vi "DeleteOneRecordTo2DListCtrl.vi"(11 "testcaselist in":refnum<vi>) -> (1 "IsEmpty?":bool, 2 "index of del":i32, 3 "testcaselist out":refnum<vi>)   [LabVIEW 2018, in "Library-Ctrl.lvlib"]
uses:
  Library-Ctrl.lvlib
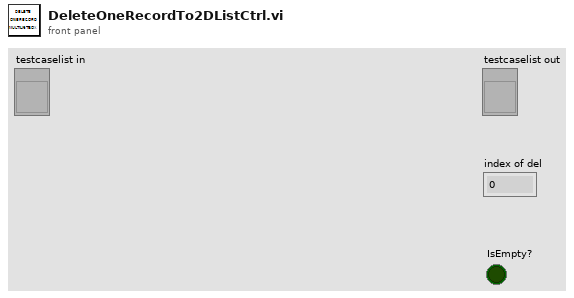
[diagram p1: front panel]
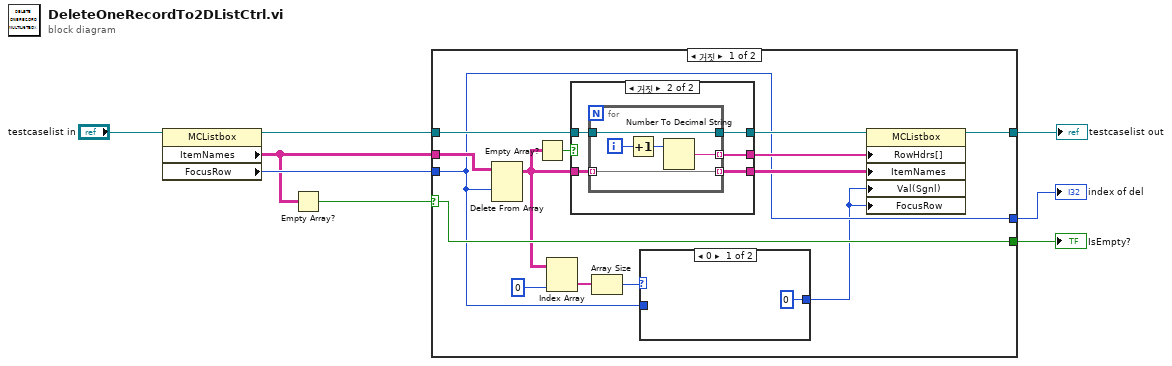
[diagram p0: block diagram]
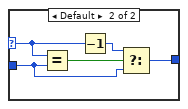
[diagram p2: hidden frame]
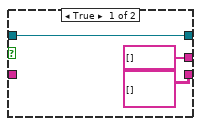
[diagram p3: hidden frame]
diagram:
  n1 = property class="MCListbox"(reference="testcaselist in") -> (reference out=w6:refnum<vi>, "ItemNames"=w4:string[][], "FocusRow"=w5:i32)  [unwired: 1 in, 1 out]
  n2 = Empty Array?(array=w4) -> (empty?=w7:bool)
  n3 = case shown="거짓" w7 {
    selector: w7 -> [w15 w43]
    tunnel: w6 -> [w18 w44]
    tunnel: w5 -> [w10 w42]
    tunnel: w4 -> [w22 _]
    tunnel: [w17 w44] -> w3
    tunnel: [w15 w43] -> w2
    tunnel: [w10 w42] -> w1
    frame False {
      n4 = Delete From Array(array=w22, index (row)=w10) -> (array with subset deleted=w14:string[][])  [unwired: 2 in, 1 out]
      n5 = Empty Array?(array=w14) -> (empty?=w16:bool)
      n6 = Index Array(array=w14, index (col)=0 ("비활성화된 인덱스 (열)")) -> (element=w12:string[])  [unwired: 1 in]
      n7 = case shown="거짓" w16 {
        tunnel: [w29 w36] -> w21
        tunnel: [string[] [] w35] -> w20
        tunnel: [string[][] [] ("ItemNames") w34] -> w19
        tunnel: w18 -> [w29 w33]
        tunnel: w14 -> [_ w32]
        frame True {
        }
        frame False {
          n8 = for {
            tunnel: w33 -> [w41]
            tunnel: [w41] -> w36
            tunnel: [w38] -> w35 mode=indexing
            tunnel: [w37] -> w34 mode=indexing
            tunnel: w32 -> [w37] mode=indexing
            i -> [w40]
            n9 = Increment(x=w40) -> (x+1=w39:i32)
            n10 = Number To Decimal String(number=w39) -> (decimal integer string=w38:string)  [unwired: 1 in]
          }
        }
      }
      n11 = Array Size(array=w12) -> (size(s)=w11:i32)
      n12 = case shown="0" w11 {
        selector: w11 -> [_ w27]
        tunnel: w10 -> [_ w25]
        tunnel: [0 ("FocusRow") w24] -> w9
        frame 0 {
        }
        frame Default {
          n13 = Equal?(x=w27, y=w25) -> (x = y?=w28:bool)
          n14 = Decrement(x=w27) -> (x-1=w26:i32)
          n15 = Select(t=w26, s=w28, f=w25) -> (s? t:f=w24:i32)
        }
      }
      n16 = property class="MCListbox"(reference=w21, "RowHdrs[]"=w20, "ItemNames"=w19, "Val(Sgnl)"=w9, "FocusRow"=w9) -> (reference out=w17:refnum<vi>)  [unwired: 1 in, 1 out]
    }
    frame True {
    }
  }
  "testcaselist out" <- w3
  "IsEmpty?" <- w2
  "index of del" <- w1
